vi "DestroyEvents.vi"(8 "error in (no error)":errorcluster, 11 "TestApplication in":refnum<class "TestApplication.lvclass">) -> (0 "error out":errorcluster, 3 "TestApplication out":refnum<class "TestApplication.lvclass">)   [LabVIEW 2022 SP3, in "Demo.lvlib" / "TestApplication.lvclass"]
uses:
  TestApplication.lvclass
  TestApplication.lvclass/TestApplication.ctl
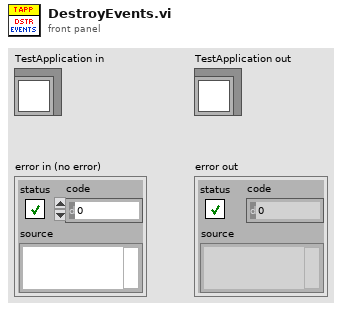
[diagram p1: front panel]
types:
  T1 = typedef "Demo.lvlib/TestApplication.lvclass/_Events.ctl" = cluster{"ToggleLed":refnum<user-event>}
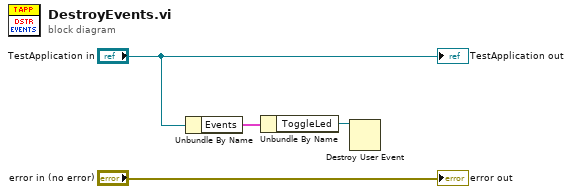
[diagram p0: block diagram]
diagram:
  n1 = Unbundle By Name("TestApplication in") -> ("Events"=w2:T1)
  n2 = Unbundle By Name(w2) -> ("ToggleLed"=w1:refnum<user-event>)
  n3 = Destroy User Event(user event=w1) -> ()  [unwired: 1 in, 1 out]
  "error out" <- "error in (no error)"
  "TestApplication out" <- "TestApplication in"
